vi "CloseSystemDefinitionReferences.vi"(8 "error in":errorcluster, 10 "Delete Sysdef? (F)":bool, 11 "VeriStandScriptingTestCase in":refnum<class "VeriStandScriptingTestCase.lvclass">) -> (0 "error out":errorcluster, 3 "VeriStandScriptingTestCase out":refnum<class "VeriStandScriptingTestCase.lvclass">)   [LabVIEW 2027, in "VeriStandScriptingTestCase.lvclass"]
uses:
  VeriStandScriptingTestCase.lvclass
  VeriStandScriptingTestCase.lvclass/VeriStandScriptingTestCase.ctl
  C:/NetCoreDLL/NationalInstruments.VeriStand.SystemDefinitionAPI.dll
  NetCoreDLL/NationalInstruments.VeriStand.SystemDefinitionAPI.dll
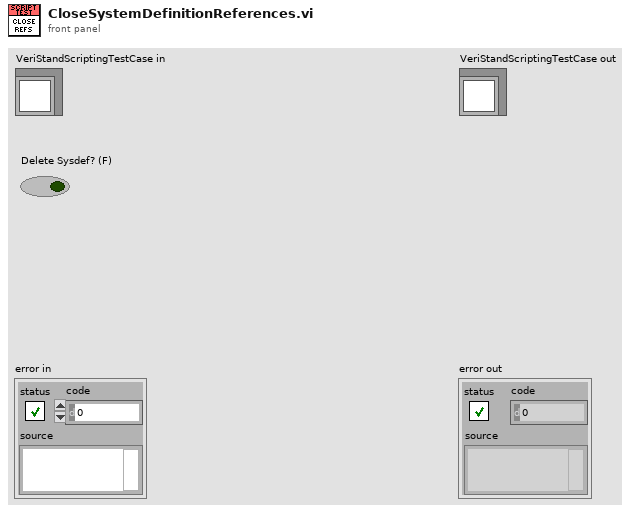
[diagram p1: front panel]
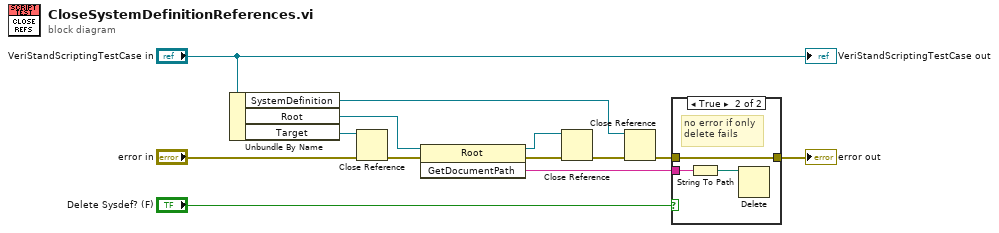
[diagram p0: block diagram]
diagram:
  n1 = Unbundle By Name("VeriStandScriptingTestCase in") -> ("SystemDefinition"=w9:refnum<k39>, "Root"=w7:refnum<k39>, "Target"=w10:refnum<k39>)
  n2 = Close Reference(reference=w10, error in (no error)="error in") -> (error out=w8:errorcluster)
  n3 = invoke class="Root" method="GetDocumentPath"(reference=w7, error in=w8) -> (reference out=w6:refnum<k39>, error out=w5:errorcluster, "GetDocumentPath"=w1:string)  [unwired: 1 in]
  n4 = Close Reference(reference=w6, error in (no error)=w5) -> (error out=w11:errorcluster)
  n5 = Close Reference(reference=w9, error in (no error)=w11) -> (error out=w3:errorcluster)
  n6 = case shown="True" "Delete Sysdef? (F)" {
    tunnel: w3 -> [w14 w15]
    tunnel: [w14 w15] -> w2
    tunnel: w1 -> [_ w17]
    frame False {
    }
    frame True {
      # "no error if only\ndelete fails"
      n7 = String To Path(string=w17) -> (path=w16:path)
      n8 = Delete(path (use dialog)=w16) -> ()  [unwired: 4 in, 3 out]
    }
  }
  "error out" <- w2
  "VeriStandScriptingTestCase out" <- "VeriStandScriptingTestCase in"
